vi "Configure Input Timer.vi"(8 "error in (no error)":errorcluster, 9 "Enable Timed Input (F: False)":bool, 10 "Timer Delay (1)":i32=1 min=0 max=60000 step=1, 11 "VISA resource name":refnum<visa-resource-name>) -> (0 "error out":errorcluster, 3 "VISA resource name out":refnum<visa-resource-name>)   [LabVIEW 2018, in "BK Precision 8600 Series.lvlib"]
doc: "Configures input timer, which will enable input for the length of a specified timer delay."
uses:
  <instrlib>/BK Precision 8600 Series/BK Precision 8600 Series.lvlib
panel:
  # "s"
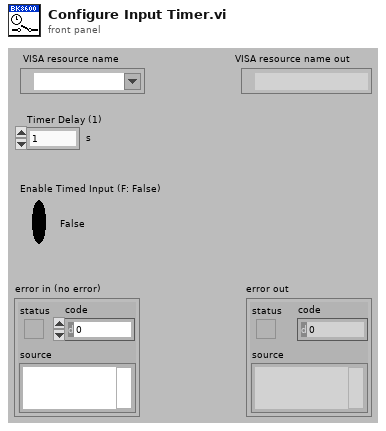
[diagram p1: front panel]
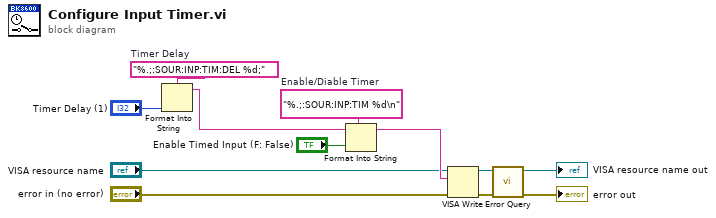
[diagram p0: block diagram]
diagram:
  w10 = "%.;:SOUR:INP:TIM %d\n"  # Enable/Diable Timer
  w12 = "%.;:SOUR:INP:TIM:DEL %d;"  # Timer Delay
  n1 = Format Into String(format string=w12, "Timer Delay (1)") -> (resulting string=w5:string)  [unwired: 2 in, 1 out]
  n2 = Format Into String(format string=w10, initial string=w5, "Enable Timed Input (F: False)") -> (resulting string=w8:string)  [unwired: 1 in, 1 out]
  n3 = VISA Write(VISA resource name="VISA resource name", write buffer=w8, error in (no error)="error in (no error)") -> (VISA resource name out=w4:refnum<visa-resource-name>, error out=w3:errorcluster)  [unwired: 1 out]
  n4 = call <instrlib>:"Error Query.vi"("error in (no error)"=w3, "VISA resource name"=w4) -> ("error out"=→"error out":errorcluster, "VISA resource name out"=→"VISA resource name out":refnum<visa-resource-name>)  [unwired: 6 in, 2 out]
